vi "Set Ring Strings and Values by Table.vi"(8 "error in (no error)":errorcluster, 10 "String and Values":string[][](table), 11 "Ring Field in":refnum<class "Ring Field.lvclass">) -> (0 "error out":errorcluster, 3 "Ring Field out":refnum<class "Ring Field.lvclass">)   [LabVIEW 2020, in "Old Basic Fields.lvlib" / "Ring Field.lvclass"]
uses:
  Ring Field.lvclass
  Old Basic Fields.lvlib
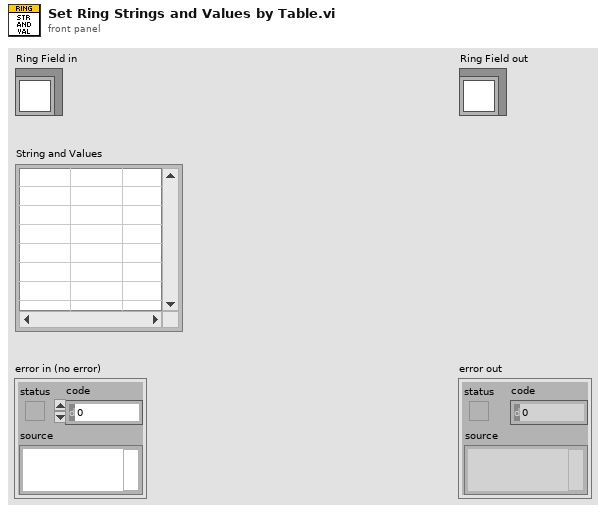
[diagram p1: front panel]
types:
  T1 = typedef "LVStringsAndValuesArrayTypeDef.ctl" = cluster{"String":string, "Value":ext}[]
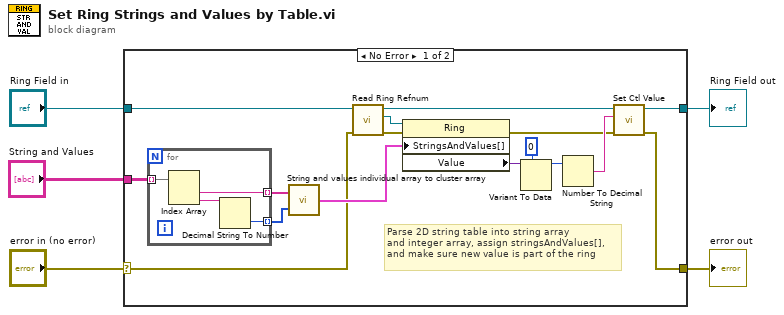
[diagram p0: block diagram]
diagram:
  n1 = case shown="No Error" "error in (no error)" {
    selector: "error in (no error)" -> [w7 w27]
    tunnel: [w6 w27] -> w4
    tunnel: [w10 w26] -> w2
    tunnel: "Ring Field in" -> [w21 w26]
    tunnel: "String and Values" -> [w18 _]
    frame No Error {
      # "Parse 2D string table into string array\nand integer array, assign stringsAndValues[],\nand make sure new value is part of the ring"
      n2 = for {
        tunnel: w18 -> [w25] mode=indexing
        tunnel: [w22] -> w13 mode=indexing
        tunnel: [w23] -> w17 mode=indexing
        n3 = Index Array(array=w25) -> (element #1=w23:string, element #2=w24:string)  [unwired: 2 in]
        n4 = Decimal String To Number(string=w24) -> (number=w22:i32)  [unwired: 2 in, 1 out]
      }
      n5 = call "String and values individual array to cluster array.vi"("Value Array In"=w13, "String Array In"=w17) -> ("Strings and Values Out"=w16:T1)
      n6 = call "Read Ring Refnum.vi"("error in (no error)"=w7, "Ring Field in"=w21) -> ("error out"=w19:errorcluster, "Ring Refnum"=w20:refnum<vi>, "Ring Field out"=w11:refnum<class "Ring Field.lvclass">)  [unwired: 7 in]
      n7 = property class="Ring"(reference=w20, error in=w19, "StringsAndValues[]"=w16) -> (error out=w8:errorcluster, "Value"=w15:variant)  [unwired: 1 out]
      n8 = Variant To Data(type=0, Variant=w15) -> (data=w12:i32)  [unwired: 1 in, 1 out]
      n9 = Number To Decimal String(number=w12) -> (decimal integer string=w9:string)  [unwired: 1 in]
      n10 = call-dynamic "Set Ctl Value.vi"("error in (no error)"=w8, "String"=w9, "Ring Field in"=w11) -> ("error out"=w6:errorcluster, "Ring Field out"=w10:refnum<class "Ring Field.lvclass">)  [unwired: 7 in]
    }
    frame Error {
    }
  }
  "error out" <- w4
  "Ring Field out" <- w2
